vi "生成2和4.vi"(10 "索引数组":cluster{"行":i32, "列":i32}[](array[cluster]), 11 "2048输入":i32[][](array[numeric])) -> (3 "2048输出":i32[][](array[numeric]))   [LabVIEW 2013]
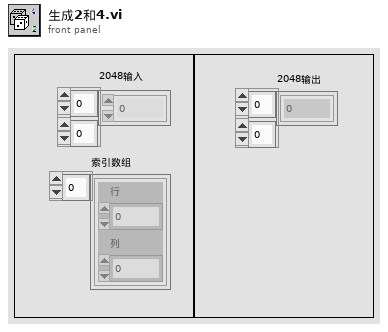
[diagram p1: front panel]
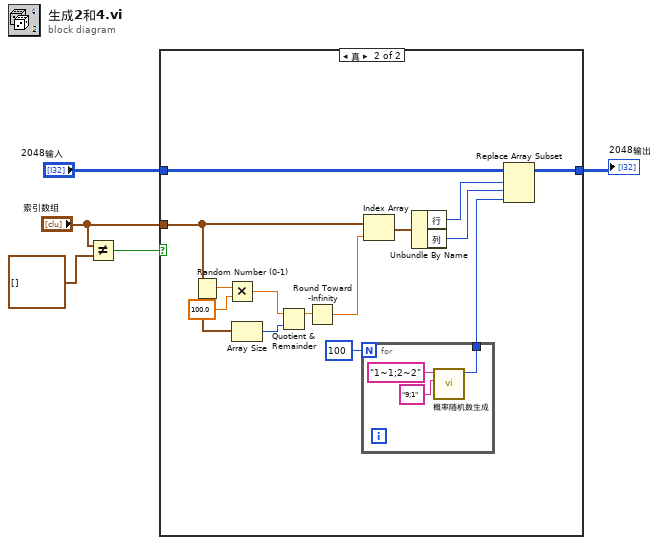
[diagram p0: block diagram]
diagram:
  n1 = Not Equal?(x="索引数组", y=cluster{"行":i32, "列":i32}[] []) -> (x != y?=w1:bool)
  n2 = case shown="真" w1 {
    tunnel: "2048输入" -> [w6 w14]
    tunnel: [w6 w9] -> w4
    tunnel: "索引数组" -> [_ w7]
    frame False {
    }
    frame True {
      n3 = Random Number (0-1)() -> (number: 0 to 1=w20:dbl)
      n4 = Multiply(x=w20, y=100.0) -> (x*y=w17:dbl)
      n5 = Array Size(array=w7) -> (size(s)=w18:i32)
      n6 = Quotient & Remainder(x=w17, y=w18) -> (x-y*floor(x/y)=w16:dbl)  [unwired: 1 out]
      n7 = Round Toward -Infinity(1:w16) -> (0:w15:dbl)
      n8 = for {
        N: 100 -> [_]
        tunnel: [w21] -> w10
        n9 = call "概率随机数生成.vi"("数值比例"="9;1", "数值范围"="1~1;2~2") -> ("整数"=w21:i32)  [unwired: 6 in, 3 out]
      }
      n10 = Index Array(array=w7, index=w15) -> (element=w13:cluster{"行":i32, "列":i32})
      n11 = Unbundle By Name(w13) -> ("行"=w12:i32, "列"=w11:i32)
      n12 = Replace Array Subset(array=w14, new element=w10, index (row)=w12, index (col)=w11) -> (w9:i32[][])
    }
  }
  "2048输出" <- w4
